vi "DAC_set_slot-jump.vi"(8 "JumpTo":T1 max=4095, 10 "slot number":u16, 11 "FPGA VI Reference In":T2) -> (3 "FPGA VI Reference Out":T2)   [LabVIEW 2013]
uses:
  fpga-bitfile-ref.ctl
  sequence slot/jump.ctl
  slot-use-values.ctl
  slot-use-type.ctl
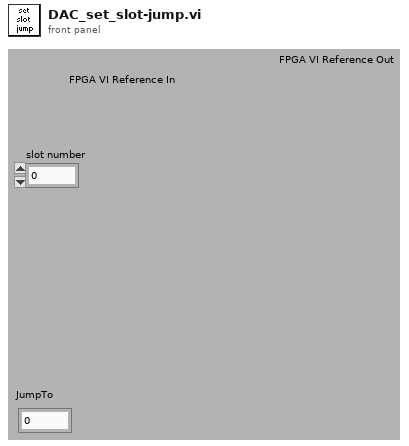
[diagram p1: front panel]
types:
  T1 = typedef "jump.ctl" = u16
  T2 = typedef "fpga-bitfile-ref.ctl" = refnum<k20>
  T3 = typedef "slot-use-type.ctl" = fxp<+,4,4>
  T4 = typedef "slot-use-values.ctl" = enum16{"DAC", "timing", "triggers", "jump"}
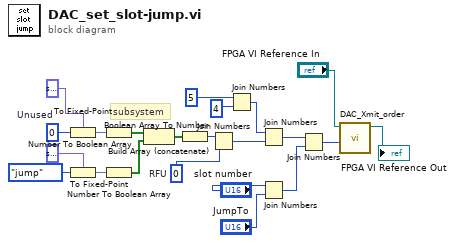
[diagram p0: block diagram]
diagram:
  w7 = u8 0  # Unused
  w3 = u8 0  # RFU
  # "subsystem"
  n1 = To Fixed-Point(fixed-point type=T3 0.0, number=w7) -> (fixed-point=w12:T3)
  n2 = To Fixed-Point(fixed-point type=T3 0.0, number=slot-use-values."jump") -> (fixed-point=w11:T3)
  n3 = Number To Boolean Array(number=w12) -> (Boolean array=w1:bool[])
  n4 = Number To Boolean Array(number=w11) -> (Boolean array=w2:bool[])
  n5 = Build Array (concatenate)(w1, w2) -> (w13:bool[])
  n6 = Boolean Array To Number(Boolean array=w13) -> (number=w4:u8)
  n7 = Join Numbers(hi=w4, lo=w3) -> ((hi.lo)=w19:u16)
  n8 = Join Numbers(hi=u8 5, lo=u8 4) -> ((hi.lo)=w18:u16)
  n9 = Join Numbers(hi=w18, lo=w19) -> ((hi.lo)=w15:u32)
  n10 = Join Numbers(hi="slot number", lo="JumpTo") -> ((hi.lo)=w16:u32)
  n11 = Join Numbers(hi=w15, lo=w16) -> ((hi.lo)=w22:u64)
  n12 = call "DAC_Xmit_order.vi"("Order in"=w22, "FPGA VI Reference In"="FPGA VI Reference In") -> ("FPGA VI Reference Out"=→"FPGA VI Reference Out":T2)  [unwired: 9 out]
